vi "morse_to_text.vi"(5 "next word":bool, 7 "next letter":bool, 8 "message in":string, 11 "buffer in":string) -> (0 "message out":string, 3 "buffer out":string)   [LabVIEW 2024]
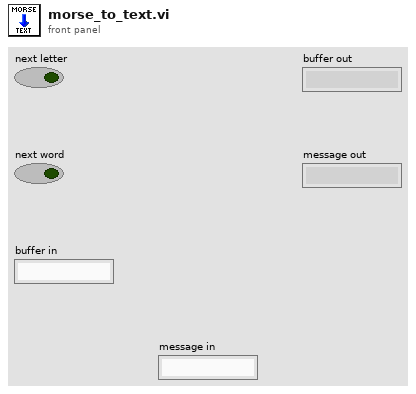
[diagram p1: front panel]
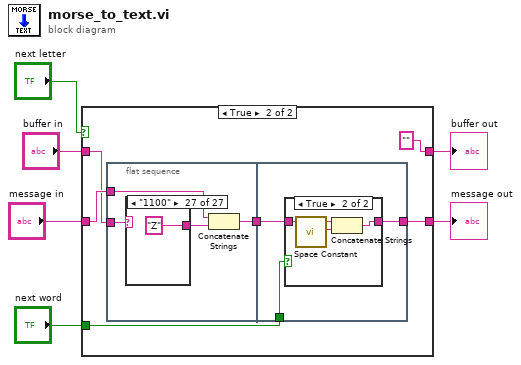
[diagram p0: block diagram]
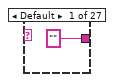
[diagram p3: hidden frame]
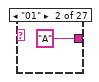
[diagram p4: hidden frame]
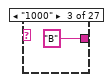
[diagram p5: hidden frame]
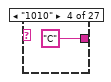
[diagram p6: hidden frame]
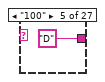
[diagram p7: hidden frame]
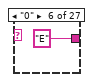
[diagram p8: hidden frame]
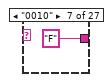
[diagram p9: hidden frame]
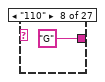
[diagram p10: hidden frame]
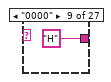
[diagram p11: hidden frame]
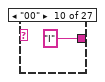
[diagram p12: hidden frame]
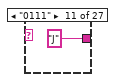
[diagram p13: hidden frame]
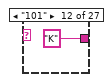
[diagram p14: hidden frame]
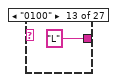
[diagram p15: hidden frame]
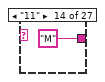
[diagram p16: hidden frame]
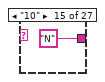
[diagram p17: hidden frame]
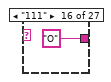
[diagram p18: hidden frame]
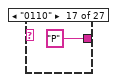
[diagram p19: hidden frame]
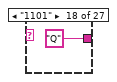
[diagram p20: hidden frame]
diagram:
  n1 = case shown="True" "next letter" {
    tunnel: "next word" -> [_ w12]
    tunnel: "message in" -> [w7 w14]
    tunnel: "buffer in" -> [w8 w11]
    tunnel: [w8 ""] -> w5
    tunnel: [w7 w9] -> w4
    frame False {
    }
    frame True {
      n2 = flat-sequence {
        tunnel: w11 -> [w18]
        tunnel: w14 -> [w17]
        tunnel: [w15] -> w13
        tunnel: w13 -> [w47]
        tunnel: w12 -> [w48]
        tunnel: [w46] -> w9
        frame #0 {
          n3 = case shown="\"1100\"" w18 {
            tunnel: ["" "A" "B" "C" "D" "E" "F" "G" "H" "I" "J" "K" "L" "M" "N" "O" "P" "Q" "R" "S" "T" "U" "V" "W" "X" "Y" "Z"] -> w16
            frame Default {
            }
            frame "01" {
            }
            frame "1000" {
            }
            frame "1010" {
            }
            frame "100" {
            }
            frame "0" {
            }
            frame "0010" {
            }
            frame "110" {
            }
            frame "0000" {
            }
            frame "00" {
            }
            frame "0111" {
            }
            frame "101" {
            }
            frame "0100" {
            }
            frame "11" {
            }
            frame "10" {
            }
            frame "111" {
            }
            frame "0110" {
            }
            frame "1101" {
            }
            frame "010" {
            }
            frame "000" {
            }
            frame "1" {
            }
            frame "001" {
            }
            frame "0001" {
            }
            frame "011" {
            }
            frame "1001" {
            }
            frame "1011" {
            }
            frame "1100" {
            }
          }
          n4 = Concatenate Strings(w17, w16) -> (w15:string)
        }
        frame #1 {
          n5 = case shown="True" w48 {
            tunnel: w47 -> [w49 w50]
            tunnel: [w49 w52] -> w46
            frame False {
            }
            frame True {
              n6 = call <vilib>:"Space Constant.vi"() -> ("String"=w51:string)
              n7 = Concatenate Strings(w50, w51) -> (w52:string)
            }
          }
        }
      }
    }
  }
  "buffer out" <- w5
  "message out" <- w4
